vi "DC_SN Verification.vi"(11 "Serial Numbers":string[](array[string])) -> (3 "Serial Numbers(out)":string[](array[string]))   [LabVIEW 2024]
panel:
  in  "Enter":bool
  # "Ensure all Serial Numbers are correct then press enter"
  # "If you need to change one,\n just edit it on the left"
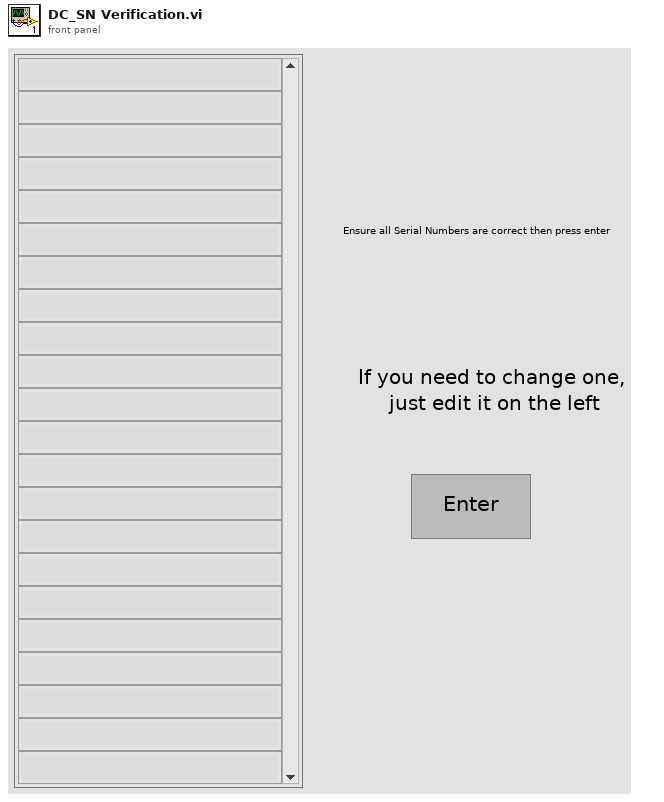
[diagram p1: front panel]
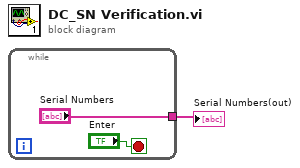
[diagram p0: block diagram]
diagram:
  n1 = while {
    tunnel: ["Serial Numbers"] -> w1
    stop <- "Enter" stop-if-true
  }
  "Serial Numbers(out)" <- w1
